vi "Move Step Tag.vi"(8 "Child tag":string, 9 "New Step Tag":string, 10 "Old Step Tag":string, 11 "TreeControl in":refnum<vi>) -> (3 "TreeControl out":refnum<vi>)   [LabVIEW 2020, in "Output Sequencer.lvlib" / "Settings UI.lvclass"]
uses:
  Settings UI.lvclass
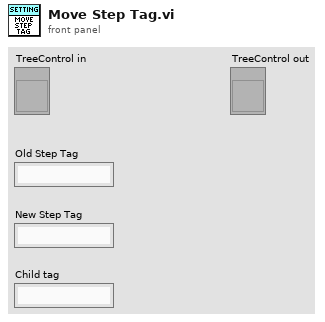
[diagram p1: front panel]
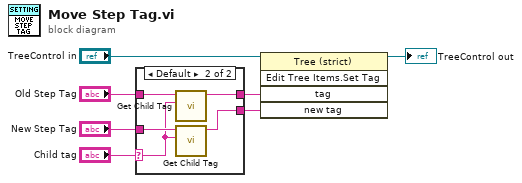
[diagram p0: block diagram]
diagram:
  n1 = case shown="Default" "Child tag" {
    selector: "Child tag" -> [_ w10]
    tunnel: [w9 w14] -> w7
    tunnel: [w8 w13] -> w6
    tunnel: "New Step Tag" -> [w8 w12]
    tunnel: "Old Step Tag" -> [w9 w11]
    frame "" {
    }
    frame Default {
      n2 = call "Get Child Tag.vi"("Child label"=w10, "Parent tag"=w11) -> ("Child tag"=w14:string)  [unwired: 9 in]
      n3 = call "Get Child Tag.vi"("Child label"=w10, "Parent tag"=w12) -> ("Child tag"=w13:string)  [unwired: 9 in]
    }
  }
  n4 = invoke class="Tree (strict)" method="Edit Tree Items.Set Tag"(reference="TreeControl in", "tag"=w7, "new tag"=w6) -> (reference out=→"TreeControl out":refnum<vi>)  [unwired: 2 in, 4 out]
